vi "Inovance_Main_Process.vi"() -> ()   [LabVIEW 2023, in "Inovance_Camera.lvlib"]
uses:
  Inovance_Camera.lvlib
  casc_correlations/ZWO/ASI_States.ctl
  <vilib>/vision/driver/NI_Vision_Acquisition_Software.lvlib
  <vilib>/userDefined/High Color/IMAQdx.ctl
  <vilib>/Utility/error.llb/DialogType.ctl
  casc_correlations/ZWO/ASI_DataCluster.ctl
  casc_correlations/Camera_Selected.ctl
  <vilib>/vision/Image Controls.llb/IMAQ Image.ctl
panel:
  out "Inovance Image":T1
  out "Error Inovance":errorcluster
  in  "Trigger Mode":enum16{"Free Run", "Hardware"}(ring)
  in  "Inovance Address":T2="Inovance_RealSpace"
  out "Inovance":bool=TRUE
  out "Inovance Reset?":bool
  in  "Live":bool
  in  "BCG Values":T3={"Brightness"=128.0, "Contrast"=45.0, "Gamma"=1.0} {"Brightness" min=0 max=255 step=1 format="%.2f"; "Contrast" min=1 max=89 step=1 format="%.2f"; "Gamma" min=0.1 max=10 step=0.01 format="%.2f"}
  in  "Exposure":dbl(slide)=3.0517578125e-05 min=3.0517578125e-05 max=1.0 step=1e-05 scale=3.2e-05..0.5
  in  "Camera Selected":T4=enum."Real Space"
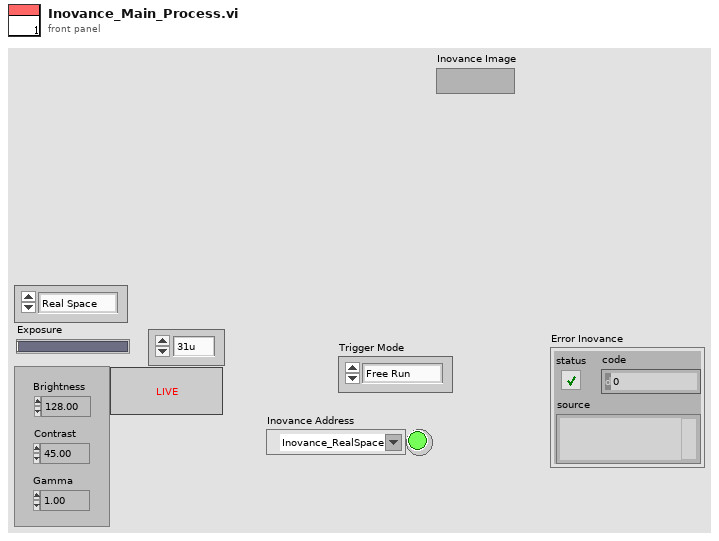
[diagram p1: front panel]
types:
  T1 = typedef "IMAQ Image.ctl" = refnum<image>
  T2 = typedef "IMAQdx.ctl" = refnum<k21>
  T3 = cluster{"Brightness":sgl, "Contrast":sgl, "Gamma":sgl}
  T4 = typedef "Camera_Selected.ctl" = enum16{"g(1)", "Real Space"}
  T5 = typedef "ASI_States.ctl" = enum16{"Init", "Idle", "Snap", "Run", "Off", "Error"}
  T6 = typedef "ASI_DataCluster.ctl" = cluster{"Gain":dbl, "Exposure":dbl, "Live":bool, "Brightness":i16}
  T7 = typedef "DialogType.ctl" = u16
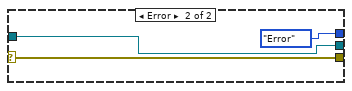
[diagram p3: hidden frame]
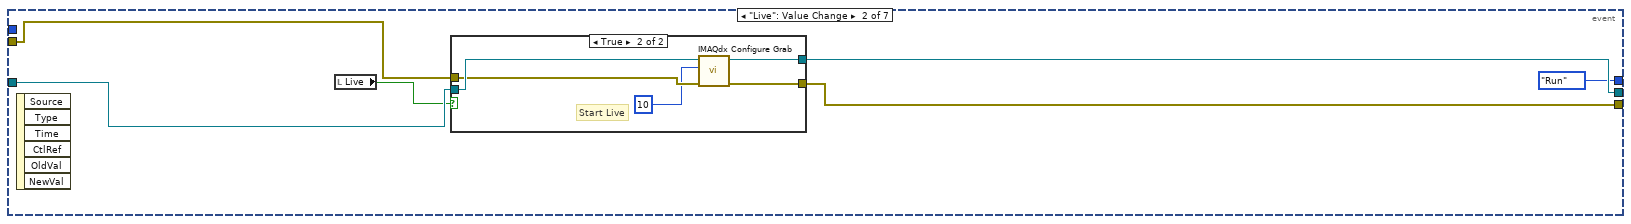
[diagram p5: hidden frame]
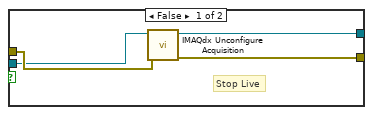
[diagram p6: hidden frame]
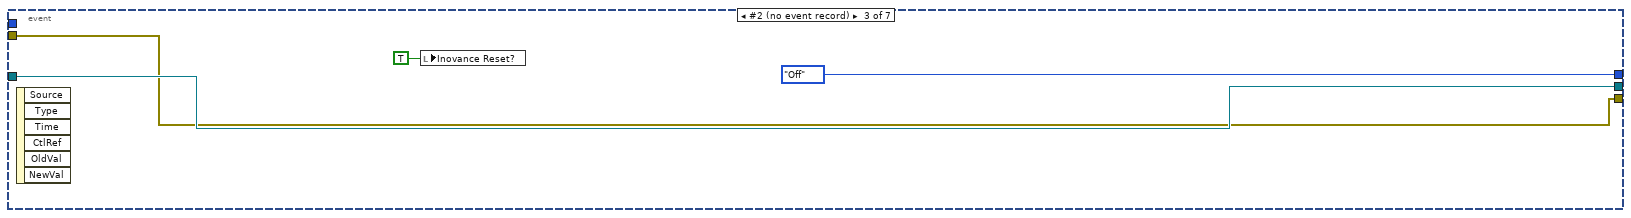
[diagram p7: hidden frame]
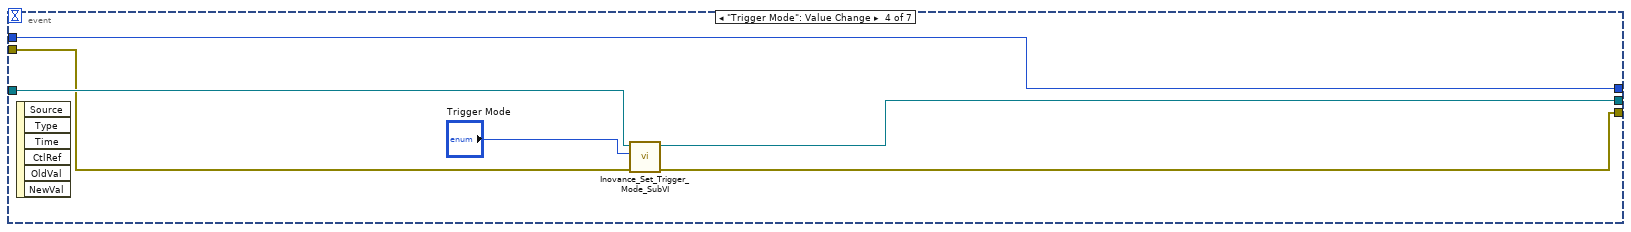
[diagram p8: hidden frame]
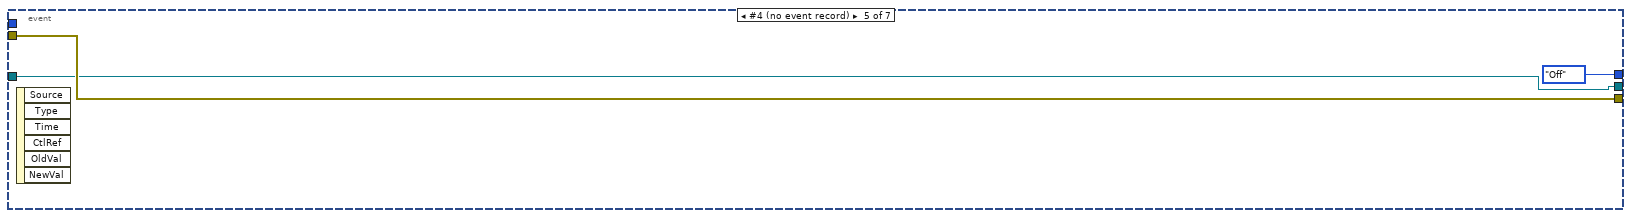
[diagram p9: hidden frame]
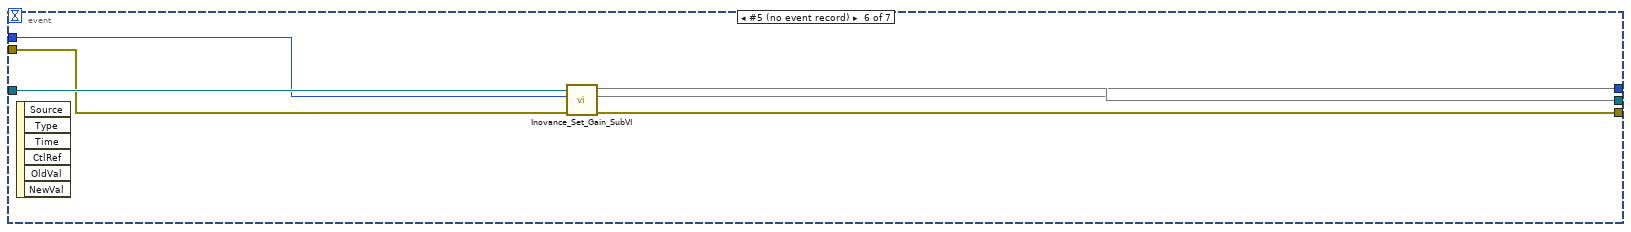
[diagram p10: hidden frame]
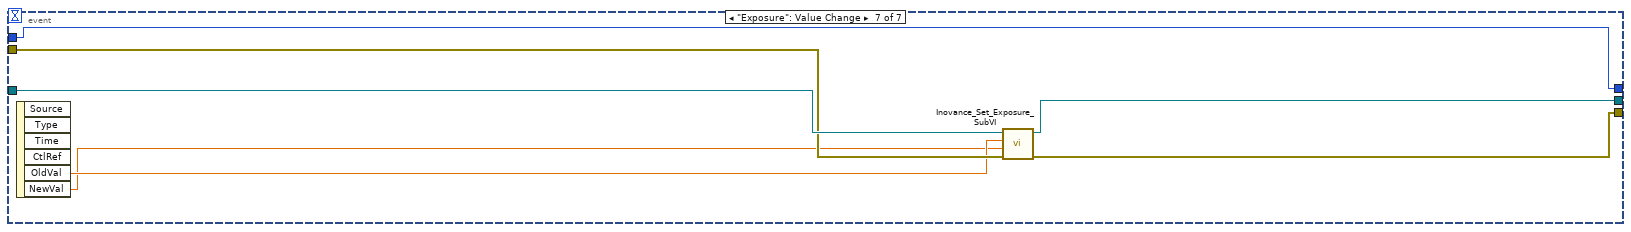
[diagram p11: hidden frame]
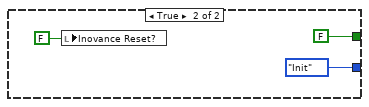
[diagram p13: hidden frame]
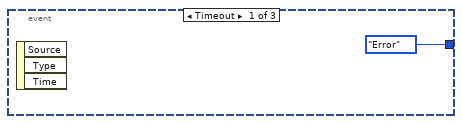
[diagram p15: hidden frame]
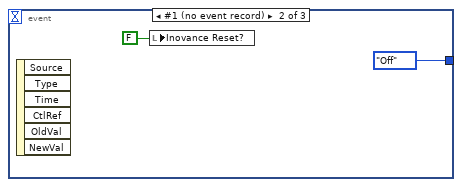
[diagram p16: hidden frame]
diagram:
  n1 = while {
    shift-right: [w5] -> _
    shift-left: ASI_States."Init" ("Array") -> [w9]
    shift-right: [w6] -> w4
    shift-left: errorcluster {"status"=FALSE, "code"=0, "source"=""} ("error in (no error)") -> [w12]
    shift-right: [w7] -> _
    shift-left: _ -> [w11]
    shift-right: [w10] -> _
    shift-left: T6 {"Gain"=0.0, "Exposure"=0.0, "Live"=FALSE, "Brightness"=0} -> [w8]
    stop <- w13 stop-if-true
    # "Inovance CMOS Process"
    n2 = case shown="\"Run\", Default" w9 {
      selector: w9 -> [_ w32 _ _]
      tunnel: w8 -> [w24 w39 w100 w111]
      tunnel: [FALSE FALSE w103 FALSE] -> w13
      tunnel: w12 -> [w23 w38 w102 w114]
      tunnel: [w20 w37 w101 errorcluster {"status"=FALSE, "code"=0, "source"=""} ("error in (no error)")] -> w6
      tunnel: [w18 w34 T2 refnum ("Session Out") w110] -> w7
      tunnel: w11 -> [_ w33 w98 w110]
      tunnel: [w24 w39 w100 w111] -> w10
      tunnel: [w19 w35 w97 w109] -> w5
      frame "Init" {
        n3 = local write "Trigger Mode"(enum16{"Free Run", "Hardware"}."Free Run" ("Trigger Mode")) -> ()
        n4 = control-ref of="Exposure"() -> ()  [unwired: 1 out]
        n5 = call "Inovance_Init_SubVI.vi"("error in (no error)"=w23) -> ("error out"=w15:errorcluster, "Refnum out"=w16:T2)  [unwired: 9 in]
        n6 = case shown="No Error" w15 {
          selector: w15 -> [w26 w29]
          tunnel: [ASI_States."Run" ("element") ASI_States."Error" ("element")] -> w19
          tunnel: w16 -> [w25 w30]
          tunnel: [w26 w29] -> w20
          tunnel: [w25 w30] -> w18
          frame No Error {
            n7 = local write "Inovance"(TRUE ("ZWO")) -> ()
          }
          frame Error {
          }
        }
        "Inovance" <- FALSE ("ZWO")
        "Inovance Reset?" <- FALSE ("ZWO Reset?")
      }
      frame "Run", Default {
        n8 = event shown="[0] Timeout" {
          selector: _ -> [_ _ _ _ _ _ _]
          dyn-events: _ -> [_ _ _ _ _ _ _]
          timeout: 50 -> [_ _ _ _ _ _ _]
          tunnel: [w43 w58 w71 w75 w82 w88 w95] -> w37
          tunnel: w38 -> [w44 w59 w71 w76 w82 w86 w93]
          tunnel: [w46 ASI_States."Run" ("Array") ASI_States."Off" ("Array") w79 ASI_States."Off" ("Array") w84 w90] -> w35
          tunnel: [w42 w57 w72 w77 w81 w85 w91] -> w34
          tunnel: w33 -> [w45 w60 w72 w78 w81 w87 w94]
          tunnel: w32 -> [w46 _ _ w79 _ w83 w90]
          event Timeout {
            n9 = event-data() -> ()  [unwired: 1 in, 3 out]
            n10 = local read "Live"() -> (w41:bool)
            n11 = case shown="True" w41 {
              tunnel: w45 -> [w48 w54]
              tunnel: [w48 w53] -> w42
              tunnel: w44 -> [w47 w52]
              tunnel: [w47 w49] -> w43
              frame False {
              }
              frame True {
                # "Grab Frame"
                n12 = local read "Inovance Image"() -> (w51:T1)
                n13 = local read "BCG Values"() -> (w50:T3)
                n14 = call "Inovance_Get_Frame_SubVI.vi"("error in (no error)"=w52, "Session Out in"=w54, "BCG Values"=w50, "Refnum in"=w51) -> ("error out"=w49:errorcluster, "Refnum out"=w53:T2)  [unwired: 6 in]
              }
            }
          }
          event "Live": Value Change {
            n15 = event-data() -> ()  [unwired: 1 in, 6 out]
            n16 = local read "Live"() -> (w55:bool)
            n17 = case shown="True" w55 {
              tunnel: w60 -> [w63 w69]
              tunnel: w59 -> [w64 w68]
              tunnel: [w62 w67] -> w57
              tunnel: [w61 w66] -> w58
              frame False {
                # "Stop Live"
                n18 = call <vilib>:"IMAQdx Unconfigure Acquisition.vi"("error in"=w64, "Session In"=w63) -> ("error out"=w61:errorcluster, "Session Out"=w62:T2)  [unwired: 8 in]
              }
              frame True {
                # "Start Live"
                n19 = call <vilib>:"IMAQdx Configure Grab.vi"("error in"=w68, "Number of Buffers"=u32 10, "Session In"=w69) -> ("error out"=w66:errorcluster, "Session Out"=w67:T2)  [unwired: 7 in]
              }
            }
          }
          event #2 (no event record) {
            n20 = event-data() -> ()  [unwired: 1 in, 6 out]
            n21 = local write "Inovance Reset?"(TRUE) -> ()
          }
          event "Trigger Mode": Value Change {
            n22 = event-data() -> ()  [unwired: 1 in, 6 out]
            n23 = call "Inovance_Set_Trigger_Mode_SubVI.vi"("error in (no error)"=w76, "Trigger Mode"="Trigger Mode", "Refnum in"=w78) -> ("error out"=w75:errorcluster, "Refnum out"=w77:T2)  [unwired: 7 in]
          }
          event #4 (no event record) {
            n24 = event-data() -> ()  [unwired: 1 in, 6 out]
          }
          event #5 (no event record) {
            n25 = event-data() -> ()  [unwired: 1 in, 6 out]
            n26 = call "Inovance_Set_Gain_SubVI.vi"("error in (no error)"=w86, 10:w83, "Refnum in"=w87) -> ("error out"=w88:errorcluster, 2:w84, 3:w85)  [unwired: 5 in, 1 out]
          }
          event "Exposure": Value Change {
            n27 = event-data() -> ("OldVal"=w92:dbl, "NewVal"=w89:dbl)  [unwired: 1 in, 4 out]
            n28 = call "Inovance_Set_Exposure_SubVI.vi"("error in (no error)"=w93, "Exposure"=w89, "OldVal"=w92, "Refnum in"=w94) -> ("error out"=w95:errorcluster, "Refnum out"=w91:T2)  [unwired: 5 in, 1 out]
          }
        }
      }
      frame "Off" {
        n29 = call <vilib>:"IMAQdx Close Camera.vi"("error in"=w102, "Session In"=w98) -> ("error out"=w101:errorcluster)  [unwired: 9 in]
        n30 = local read "Inovance Reset?"() -> (w96:bool)
        n31 = case shown="False" w96 {
          tunnel: [TRUE FALSE] -> w103
          tunnel: [ASI_States."Off" ASI_States."Init"] -> w97
          frame False {
          }
          frame True {
            n32 = local write "Inovance Reset?"(FALSE ("ZWO Reset?")) -> ()
          }
        }
      }
      frame "Error" {
        w113 = T7 0 items=["no dialog", "OK message", "continue or stop message", "OK message + warnings", "continue/stop + warnings"] ("type of dialog (OK msg:1)")
        n33 = call <vilib>:"General Error Handler.vi"("type of dialog (OK msg:1)"=w113, "error in (no error)"=w114) -> ()  [unwired: 9 in, 5 out]
        n34 = event shown="[2]" {
          selector: _ -> [_ _ _]
          dyn-events: _ -> [_ _ _]
          timeout: _ -> [_ _ _]
          tunnel: [ASI_States."Error" ASI_States."Off" ASI_States."Off"] -> w109
          event Timeout {
            n35 = event-data() -> ()  [unwired: 1 in, 3 out]
          }
          event #1 (no event record) {
            n36 = event-data() -> ()  [unwired: 1 in, 6 out]
            n37 = local write "Inovance Reset?"(FALSE) -> ()
          }
          event #2 (no event record) {
            n38 = event-data() -> ()  [unwired: 1 in, 6 out]
            n39 = local read "Inovance Reset?"() -> ()  [unwired: 1 in]
          }
        }
      }
    }
  }
  "Error Inovance" <- w4
